vi "DataBLFFileRichInfo.vi"(9 "Language":u32, 11 "file path (dialog if empty)":path caption="文件路径 （空时为对话框）") -> (0 "路径输出":path, 1 "FileInfo":string, 2 "文件类型":string)   [LabVIEW 2015]
uses:
  BLF/Read Write BLF.lvclass/Read Write BLF.ctl
  GetBinlogdllpath.vi
  BasicAppPath.vi
  <vilib>/Utility/libraryn.llb/Check if File or Folder Exists.vi
  <vilib>/Utility/error.llb/Error Cluster From Error Code.vi
  BLF/Read Write BLF.lvclass
panel:
  out "Object Count":u32
  out "总帧数":i32
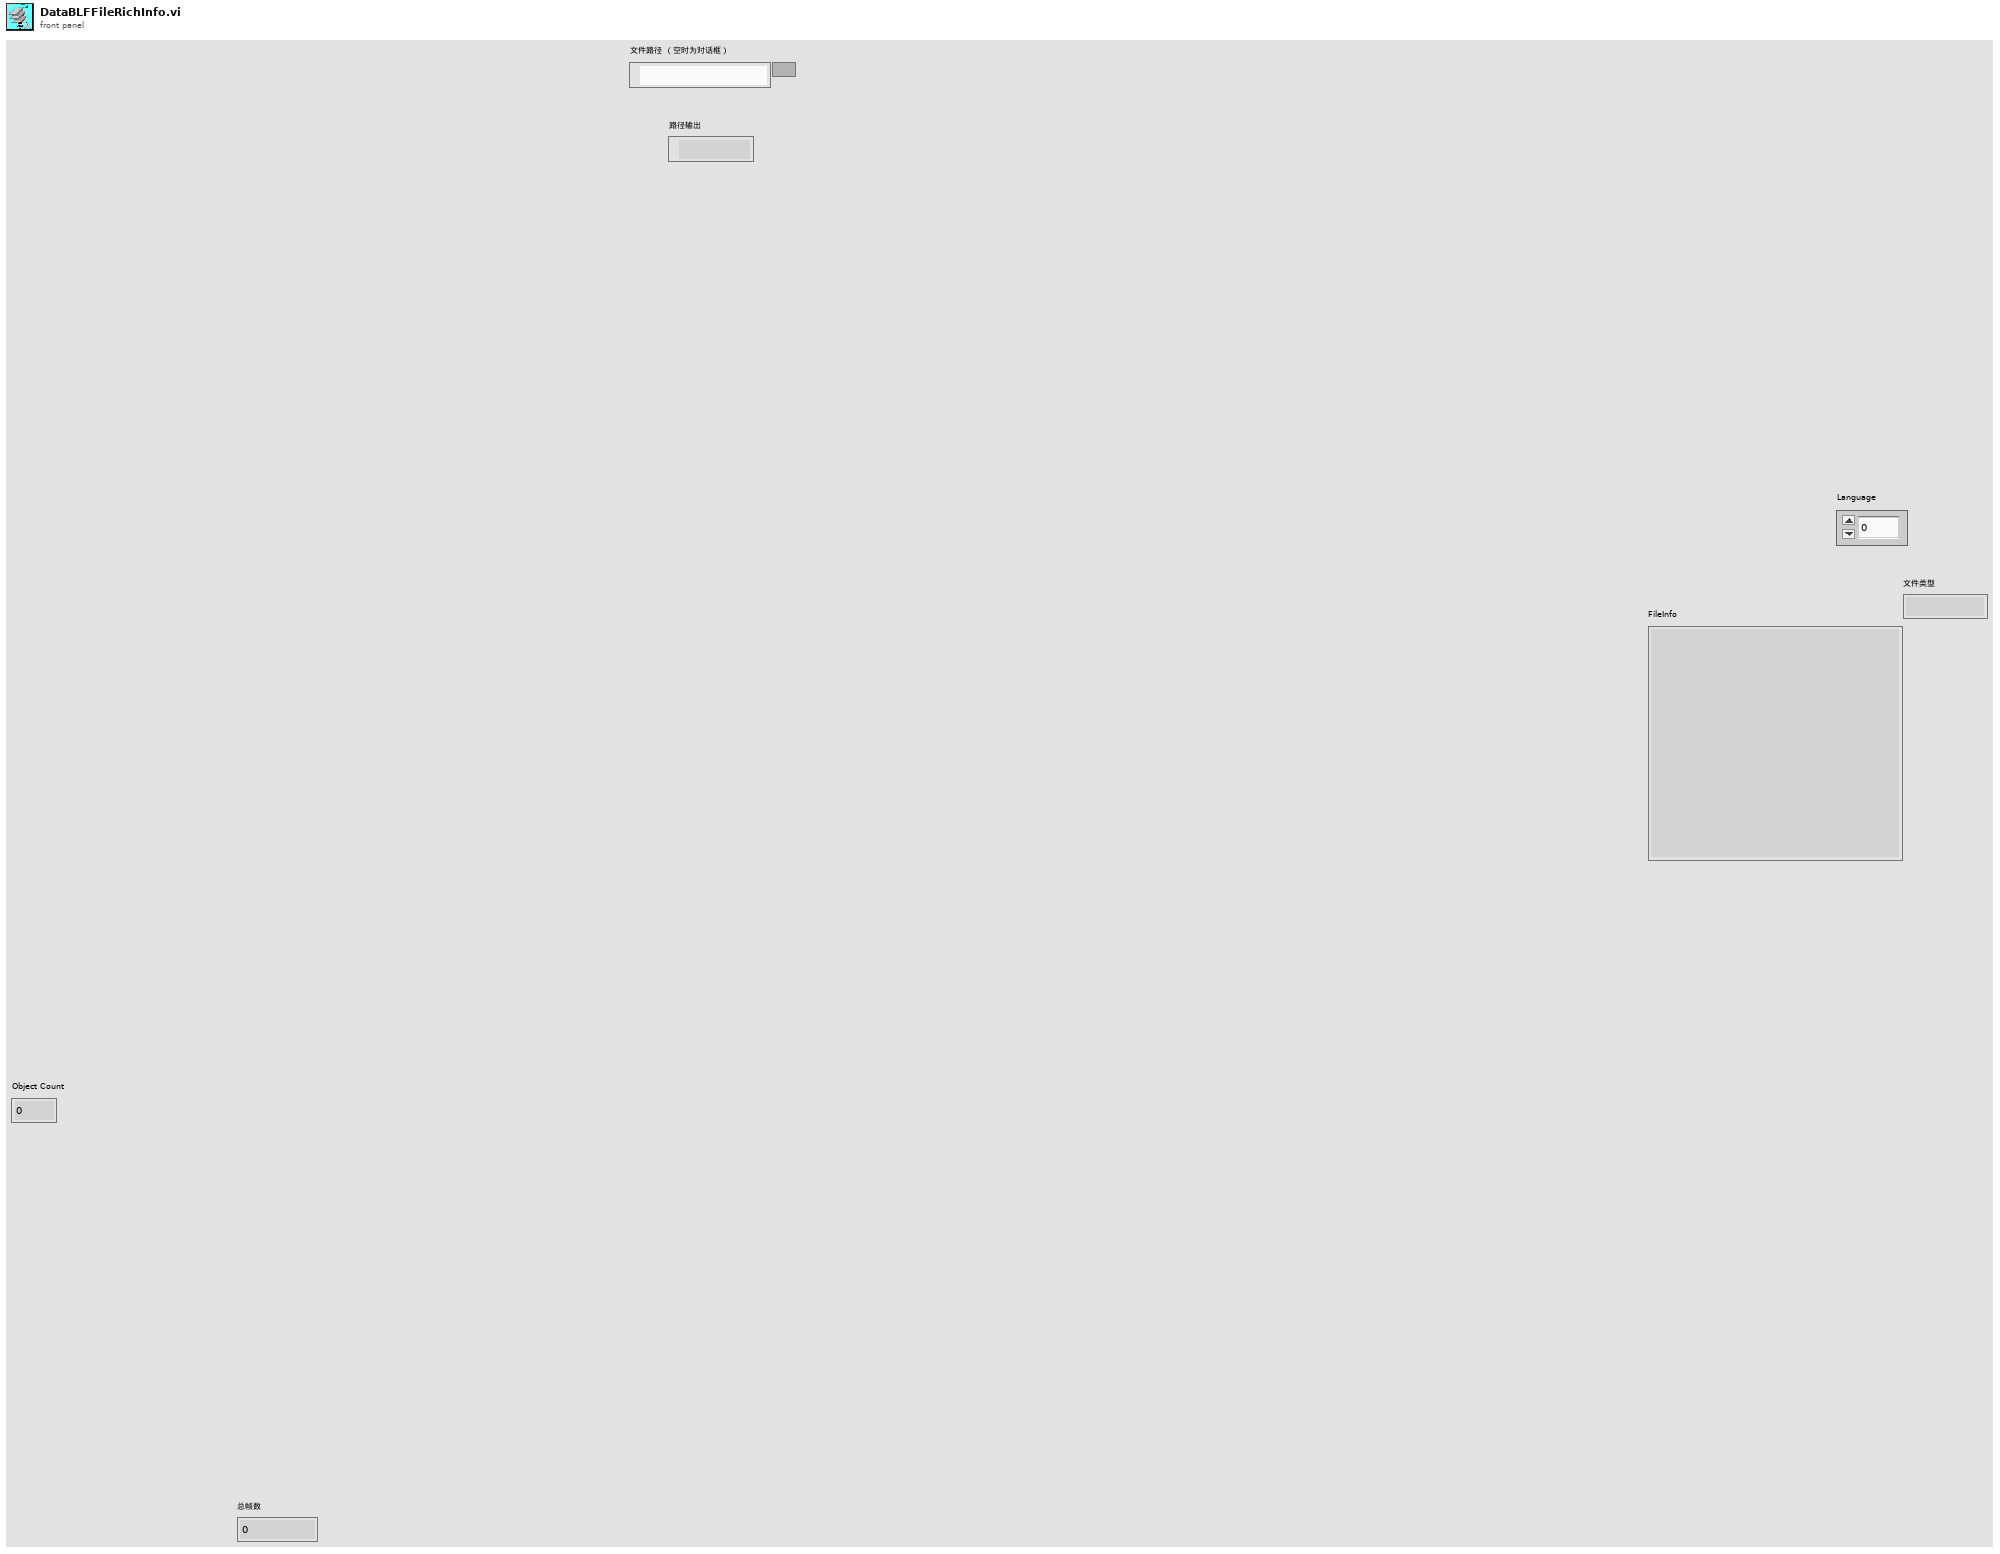
[diagram p1: front panel]
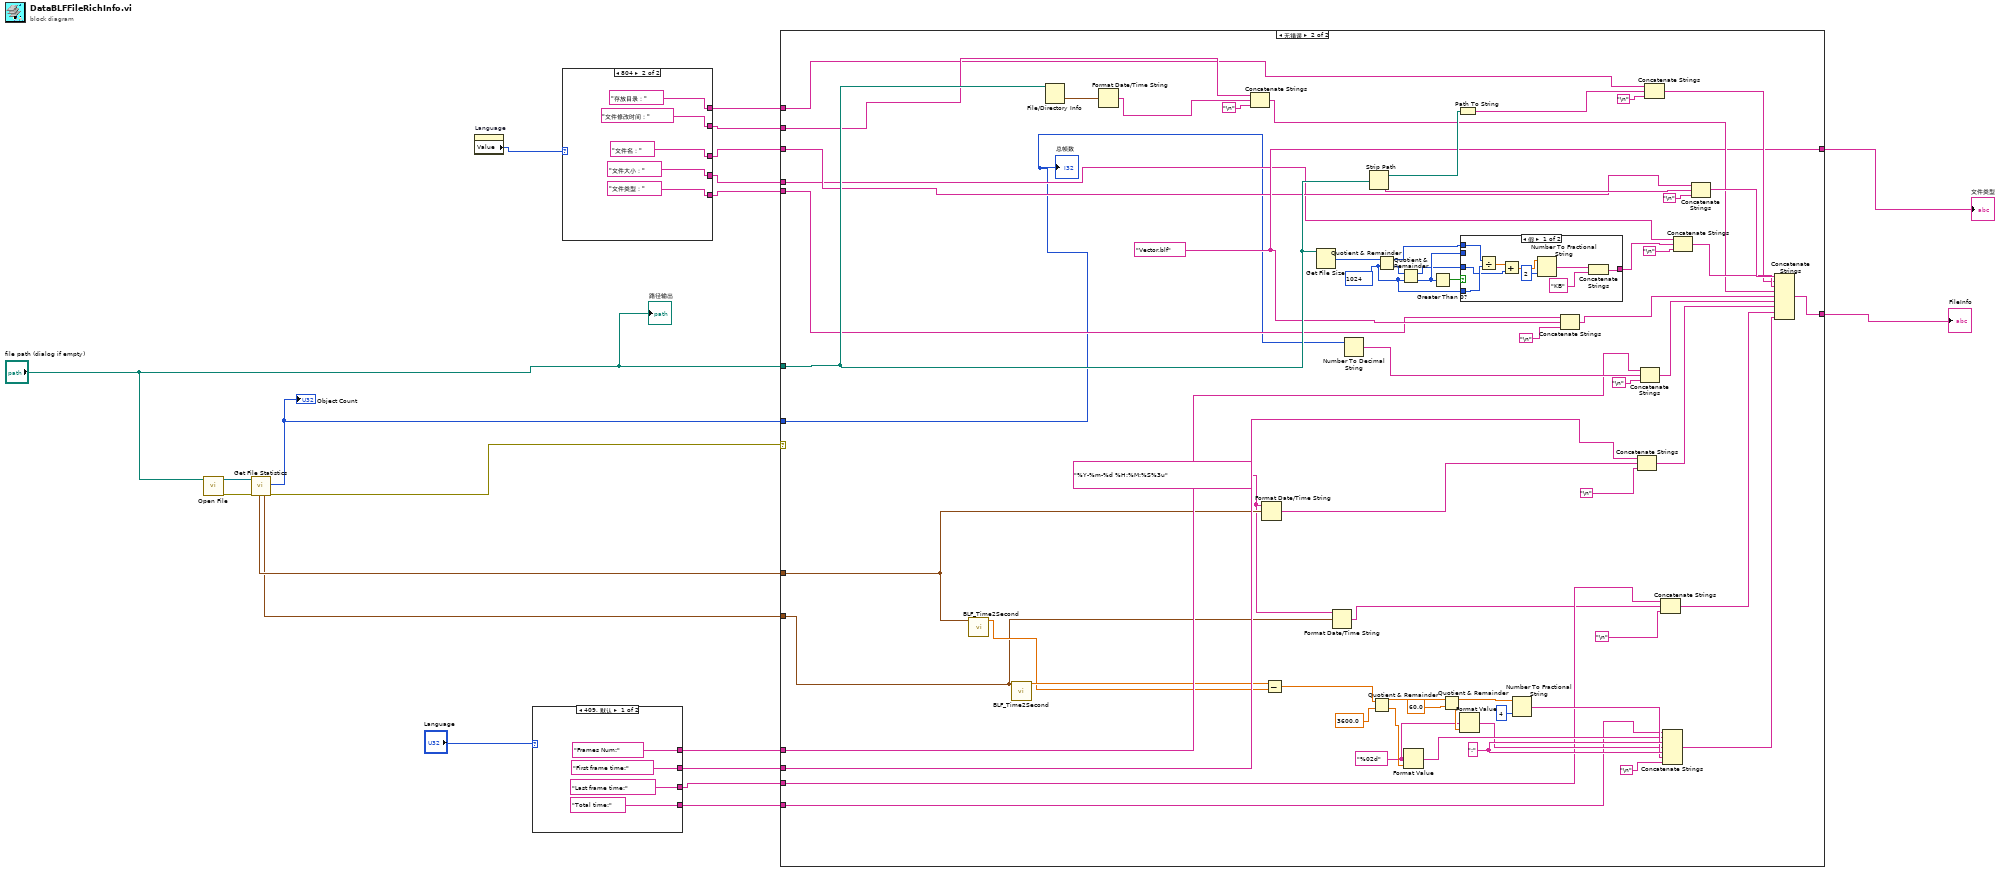
[diagram p0: block diagram]
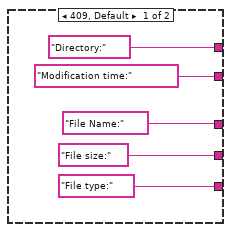
[diagram p2: hidden frame]
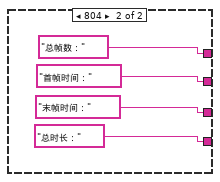
[diagram p3: hidden frame]
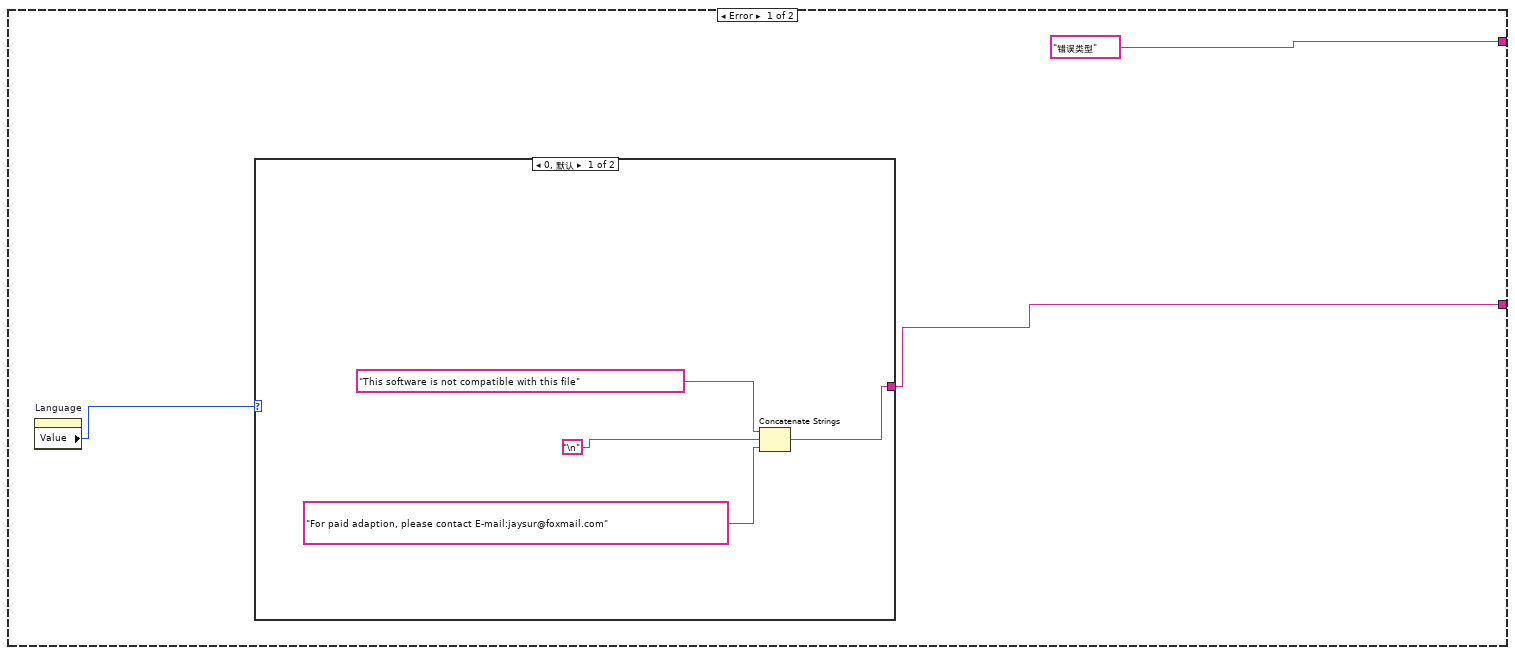
[diagram p4: hidden frame]
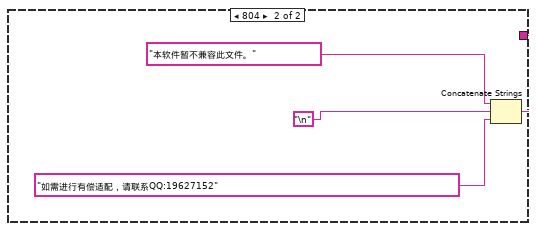
[diagram p5: hidden frame]
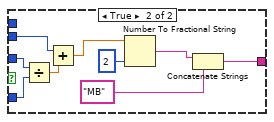
[diagram p6: hidden frame]
diagram:
  n1 = call "Open File.vi"("Log Path"="file path (dialog if empty)") -> ("error out"=w6:errorcluster, "BLF File"=w7:refnum<class "Read Write BLF.lvclass">)  [unwired: 9 in]
  n2 = call "Get File Statistics.vi"("error in (no error)"=w6, "Read Write BLF in"=w7) -> ("error out"=w4:errorcluster, "Object Count"=w3:u32, "Last Object Time"=w1:timestamp, "Start Time"=w2:timestamp)  [unwired: 3 in, 3 out]
  "Object Count" <- w3
  n3 = property on="Language" class="DigNum (严格)"() -> ("Value"=w17:u32)  [unwired: 2 in, 2 out]
  n4 = case shown="409, 默认" "Language" {
    tunnel: ["Total time:" "总时长："] -> w11
    tunnel: ["Last frame time:" "末帧时间："] -> w10
    tunnel: ["First frame time:" "首帧时间："] -> w9
    tunnel: ["Frames Num:" "总帧数："] -> w8
    frame 409, Default {
    }
    frame 804 {
    }
  }
  n5 = case shown="804" w17 {
    tunnel: ["Modification time:" "文件修改时间："] -> w16
    tunnel: ["Directory:" "存放目录："] -> w13
    tunnel: ["File Name:" "文件名："] -> w14
    tunnel: ["File size:" "文件大小："] -> w12
    tunnel: ["File type:" "文件类型："] -> w15
    frame 409, Default {
    }
    frame 804 {
    }
  }
  n6 = case shown="无错误" w4 {
    tunnel: ["错误类型" w68] -> w20
    tunnel: [w40 w114] -> w19
    tunnel: "file path (dialog if empty)" -> [_ w71]
    tunnel: w16 -> [_ w69]
    tunnel: w15 -> [_ w67]
    tunnel: w14 -> [_ w66]
    tunnel: w13 -> [_ w65]
    tunnel: w12 -> [_ w64]
    tunnel: w11 -> [_ w63]
    tunnel: w10 -> [_ w62]
    tunnel: w9 -> [_ w61]
    tunnel: w8 -> [_ w60]
    tunnel: w3 -> [_ w59]
    tunnel: w2 -> [_ w54]
    tunnel: w1 -> [_ w52]
    frame Error {
      n7 = property on="Language" class="DigNum (严格)"() -> ("Value"=w39:u32)  [unwired: 2 in, 2 out]
      n8 = case shown="0, 默认" w39 {
        tunnel: [w42 w46] -> w40
        frame 0, Default {
          n9 = Concatenate Strings("This software is not compatible with this file", "\n", "For paid adaption, please contact E-mail:jaysur@foxmail.com") -> (w42:string)
        }
        frame 804 {
          n10 = Concatenate Strings("本软件暂不兼容此文件。", "\n", "如需进行有偿适配，请联系QQ:19627152") -> (w46:string)
        }
      }
    }
    frame No Error {
      w51 = "%Y-%m-%d %H:%M:%S%3u" ("时间格式字符串(%c)")
      w68 = "Vector.blf"
      w83 = i64 1024 ("y")
      w100 = "%02d" ("格式字符串")
      w106 = ":"
      n11 = call "BLF_Time2Second.vi"("Time"=w54) -> ("Second"=w56:dbl)  [unwired: 10 in]
      n12 = call "BLF_Time2Second.vi"("Time"=w52) -> ("Second"=w57:dbl)  [unwired: 10 in]
      n13 = File/Directory Info(path=w71) -> (last mod=w74:timestamp)  [unwired: 1 in, 6 out]
      n14 = Format Date/Time String(seconds (now)=w74) -> (date/time string=w72:string)  [unwired: 2 in]
      n15 = Concatenate Strings(w69, w72, "\n") -> (w70:string)
      n16 = Format Date/Time String(time format string (%c)=w51, seconds (now)=w54) -> (date/time string=w53:string)  [unwired: 1 in]
      n17 = Subtract(x=w57, y=w56) -> (x-y=w99:dbl)
      n18 = Get File Size(file=w71) -> (size (in bytes)=w86:i64)  [unwired: 1 in, 2 out]
      n19 = Format Date/Time String(time format string (%c)=w51, seconds (now)=w52) -> (date/time string=w50:string)  [unwired: 1 in]
      n20 = Number To Decimal String(number=w59) -> (decimal integer string=w89:string)  [unwired: 1 in]
      n21 = Strip Path(path=w71) -> (stripped path=w76:path, name=w96:string)
      n22 = Quotient & Remainder(x=w99, y=3600.0) -> (x-y*floor(x/y)=w110:dbl, floor(x/y)=w103:dbl)
      n23 = Quotient & Remainder(x=w86, y=w83) -> (x-y*floor(x/y)=w79:i64, floor(x/y)=w85:i64)
      n24 = Quotient & Remainder(x=w85, y=w83) -> (x-y*floor(x/y)=w81:i64, floor(x/y)=w82:i64)
      n25 = Format Value(format string=w100, value (0)=w103) -> (output string=w104:string)  [unwired: 1 in]
      n26 = Greater Than 0?(x=w82) -> (x > 0?=w84:bool)
      n27 = Quotient & Remainder(x=w110, y=60.0) -> (x-y*floor(x/y)=w108:dbl, floor(x/y)=w102:dbl)
      n28 = Path To String(path=w76) -> (string=w77:string)
      n29 = Format Value(format string=w100, value (0)=w102) -> (output string=w101:string)  [unwired: 1 in]
      n30 = case shown="假" w84 {
        tunnel: w83 -> [w120 w130]
        tunnel: w82 -> [_ w128]
        tunnel: w81 -> [w118 w131]
        tunnel: [w123 w126] -> w80
        tunnel: w79 -> [w121 _]
        frame False {
          n31 = Divide(x=w121, y=w120) -> (x/y=w119:dbl)
          n32 = Add(x=w119, y=w118) -> (x+y=w117:dbl)
          n33 = Number To Fractional String(number=w117, precision (6)=i16 2 ("精度(6)")) -> (F-format string=w115:string)  [unwired: 2 in]
          n34 = Concatenate Strings(w115, "KB" ("字符串")) -> (w123:string)
        }
        frame True {
          n35 = Divide(x=w131, y=w130) -> (x/y=w129:dbl)
          n36 = Add(x=w128, y=w129) -> (x+y=w127:dbl)
          n37 = Number To Fractional String(number=w127, precision (6)=i16 2 ("精度(6)")) -> (F-format string=w125:string)  [unwired: 2 in]
          n38 = Concatenate Strings(w125, "MB") -> (w126:string)
        }
      }
      n39 = Number To Fractional String(number=w108, precision (6)=i16 4 ("精度(6)")) -> (F-format string=w105:string)  [unwired: 2 in]
      n40 = Concatenate Strings(w67, w68, "\n") -> (w93:string)
      n41 = Concatenate Strings(w61, w53, "\n") -> (w113:string)
      n42 = Concatenate Strings(w60, w89, "\n") -> (w90:string)
      n43 = Concatenate Strings(w65, w77, "\n") -> (w75:string)
      n44 = Concatenate Strings(w62, w50, "\n") -> (w112:string)
      n45 = Concatenate Strings(w63, w104, w106, w101, w106, w105, "\n") -> (w98:string)
      n46 = Concatenate Strings(w64, w80, "\n") -> (w87:string)
      n47 = Concatenate Strings(w66, w96, "\n") -> (w95:string)
      n48 = Concatenate Strings(w95, w75, w87, w70, w93, w90, w113, w112, w98) -> (w114:string)
      "总帧数" <- w59
    }
  }
  "FileInfo" <- w19
  "文件类型" <- w20
  "路径输出" <- "file path (dialog if empty)"
